vi "Dequeue Transport Element.vi"(8 "error in (no error)":errorcluster, 9 "Timeout In ms (-1)":i32=-1, 11 "QueueTransport in":refnum<class "QueueTransport.lvclass">) -> (0 "error out":errorcluster, 1 "Publication Time":timestamp, 2 "Data":variant, 3 "QueueTransport out":refnum<class "QueueTransport.lvclass">)   [LabVIEW 2017, in "Transport.lvlib" / "QueueTransport.lvclass"]
uses:
  QueueTransport.lvclass
  QueueTransport.lvclass/QueueTransport.ctl
  <vilib>/Utility/error.llb/Error Cluster From Error Code.vi
  <vilib>/ErrorRing/Error Ring.xnode
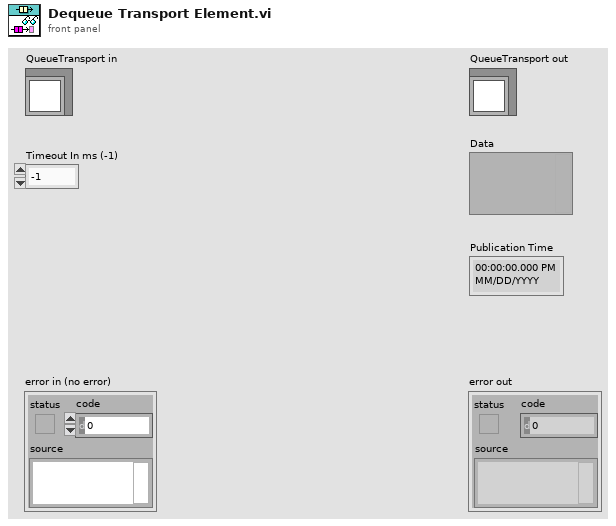
[diagram p1: front panel]
types:
  T1 = cluster{"Data":variant, "Publication Time":timestamp}
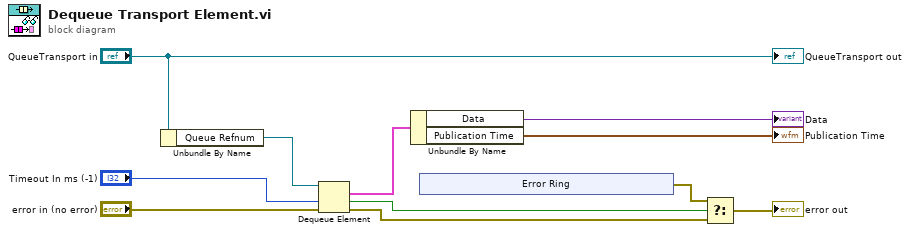
[diagram p0: block diagram]
diagram:
  n1 = Unbundle By Name("QueueTransport in") -> ("Queue Refnum"=w5:refnum<queue>)
  n2 = Dequeue Element(queue=w5, timeout in ms (-1)="Timeout In ms (-1)", error in (no error)="error in (no error)") -> (element=w8:T1, timed out?=w3:bool, error out=w2:errorcluster)  [unwired: 1 out]
  n3 = Unbundle By Name(w8) -> ("Data"=→"Data":variant, "Publication Time"=→"Publication Time":timestamp)
  n4 = xnode "Error Ring"() -> ("error out"=w1:errorcluster)
  n5 = Select(t=w1, s=w3, f=w2) -> (s? t:f=→"error out":errorcluster)
  "QueueTransport out" <- "QueueTransport in"
